vi "Flush Buffer.vi"(8 "error in (no error)":errorcluster, 10 "Wfm Log Instance Index":i32, 11 "Waveform Log in":refnum<class "Waveform Log.lvclass">) -> (0 "error out":errorcluster, 3 "Waveform Log out":refnum<class "Waveform Log.lvclass">)   [LabVIEW 2015, in "Waveform Log.lvclass"]
uses:
  Waveform Log.lvclass
  Waveform Log.lvclass/Waveform Log.ctl
  Buffer/Waveform Buffer/Time Range.ctl
  Buffer/Waveform Buffer/Waveform Buffer.lvclass/Waveform Buffer.ctl
  Waveform Log Wfm Meta Data.ctl
  Buffer/DBL Waveform Buffer/DBL Waveform Buffer.lvclass/DBL Waveform Buffer.ctl
  Logs/Segmented Logs/Segmented Log/Segmented Log.lvclass/Segmented Log.ctl
  Log File Specifications/Log File Specification/Log File Specification.lvclass/Log File Specification.ctl
  Log File Specifications/Waveform TDMS Log File Specification/Waveform TDMS Log File Specification.lvclass/Waveform TDMS Log File Specification.ctl
  Logs/Log Files/Log File/Log File.lvclass/Log File.ctl
  Logs/Log Files/TDMS Log File/TDMS Log File.lvclass/TDMS Log File.ctl
  Logs/Log Files/Text Log File/Text Log File.lvclass/Text Log File.ctl
  Logs/Segmented Logs/Footprint Segmented Log/Footprint Segmented Log.lvclass/Footprint Segmented Log.ctl
  Logs/Segmented Logs/Time Segmented Log/Time Segmented Log.lvclass/Time Segmented Log.ctl
  Buffer/Waveform Buffer/Shift Point by Time.vi
  Buffer/Waveform Buffer/Split Divided Segment.vi
  Buffer/DBL Waveform Buffer/DBL Read from Buffer.vi
  Logs/Segmented Logs/Segmented Log/Write Waveform to Log File Instance.vi
  Buffer/Waveform Buffer/Shift Point by Samples.vi
  Buffer/Waveform Buffer/Get Buffer Length.vi
  Log File Specifications/Log File Specification/Get Log Specification Type.vi
  Log File Specifications/Waveform TDMS Log File Specification/Get Current Group.vi
  Logs/Log Files/Log File/Get Log File Type.vi
  Logs/Log Files/Log File/Write Channel to Log File.vi
  Logs/Log Files/TDMS Log File/Set TDMS Channel Property.vi
  Logs/Log Files/TDMS Log File/Copy Channel Properties.vi
  Logs/Segmented Logs/Segmented Log/Check Close File.vi
  Logs/Segmented Logs/Segmented Log/Check Open File.vi
  Logs/Log Files/TDMS Log File/Write Channel to TDMS Log File.vi
  Logs/Log Files/Text Log File/Write Channel to Text Log File.vi
  Logs/Segmented Logs/Segmented Log/Close Log File Instance.vi
  Logs/Segmented Logs/Segmented Log/Segment Log File.vi
  Logs/Segmented Logs/Segmented Log/Open Log File Instance.vi
  Logs/Log Files/Log File/Close Log File.vi
  Logs/Segmented Logs/Segmented Log/Make File Read-Only.vi
  Logs/Segmented Logs/Segmented Log/On Segmented Log Complete.vi
  Logs/Segmented Logs/Segmented Log/On File Close.vi
  Logs/Segmented Logs/Footprint Segmented Log/Segment Log File (Footprint).vi
  Logs/Segmented Logs/Time Segmented Log/Segment Log File (Time).vi
  Log File Specifications/Log File Specification/Open Log File.vi
  Log File Specifications/Log File Specification/Set Path Tag.vi
  Logs/Segmented Logs/Segmented Log/On File Open.vi
  Log File Specifications/Log File Specification/Set Filename Offset.vi
  Logs/Log Files/TDMS Log File/Close TDMS Log File.vi
  Logs/Log Files/Text Log File/Close Text Log File.vi
  Logs/Segmented Logs/Segmented Log/Get Current Log File Instance.vi
  Logs/Log Files/Log File/Get File Size.vi
  Logs/Log Files/Log File/Get Start Time.vi
  Log File Specifications/Log File Specification/Build File Path.vi
  Log File Specifications/Log File Specification/Resolve File Conflicts.vi
  Shared/Utility/Format File Path for Linux.vi
  <vilib>/Utility/error.llb/Error Cluster From Error Code.vi
  Log File Specifications/Log File Specification/Initialize Log File.vi
  <vilib>/Utility/libraryn.llb/Create Directory Recursive.vi
  <vilib>/Utility/libraryn.llb/Check if File or Folder Exists.vi
  <vilib>/Utility/libraryn.llb/Get File Extension.vi
  Logs/Log Files/Text Log File/Text Log File.lvclass
  Logs/Log Files/TDMS Log File/TDMS Log File.lvclass
  Logs/Log Files/Log File/Log File.lvclass
  Logs/Segmented Logs/Time Segmented Log/Time Segmented Log.lvclass
  Logs/Segmented Logs/Footprint Segmented Log/Footprint Segmented Log.lvclass
  Log File Specifications/Waveform TDMS Log File Specification/Waveform TDMS Log File Specification.lvclass
  Buffer/DBL Waveform Buffer/DBL Waveform Buffer.lvclass
  Buffer/Waveform Buffer/Waveform Buffer.lvclass
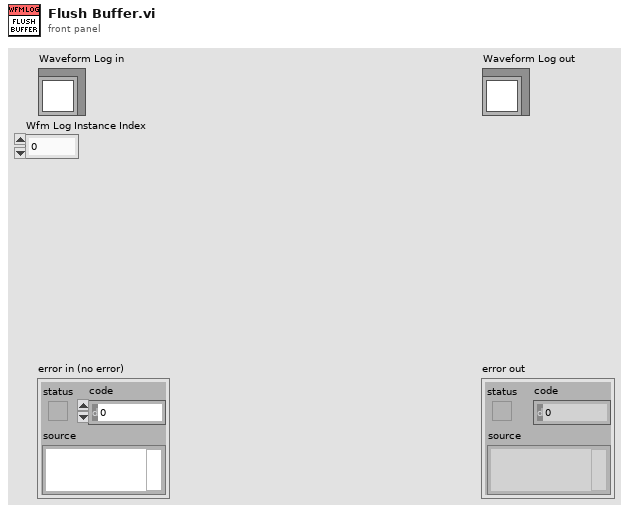
[diagram p1: front panel]
types:
  T1 = typedef "Waveform Buffer.lvclass/Time Range.ctl" = cluster{"Use Receive Time":bool, "Start Time":timestamp, "Stop time":timestamp}
  T2 = typedef "Waveform Log.lvclass/Waveform Log Wfm Meta Data.ctl" = cluster{"Segment ID":u64, "dt":dbl, "t0":timestamp, "tf":timestamp}
  T3 = typedef "Waveform Log.lvclass/Log Instance.ctl" = cluster{"Segmented Log":refnum<data-value>, "Log Waveforms":T4[], "Log Start":timestamp, "Log Stop":timestamp, "Start Trigger Time":timestamp, "Stop Trigger Time":timestamp, "Time of Last Write":timestamp, "Timeout":dbl, "Stop cmd received":bool}
  T4 = typedef "Waveform Log.lvclass/Log Instance Waveform.ctl" = cluster{"Wfm Info":T5, "Count / Instance":i32, "Previous Segment":u64, "Wfm Complete?":bool, "Last Sample Logged":timestamp, "Data Logged":bool, "Log segmented":bool}
  T5 = typedef "Waveform Log.lvclass/Waveform Information.ctl" = cluster{"Name":string, "Wfm Data Type":T6, "Decimation":u32}
  T6 = typedef "Waveform Log.lvclass/Waveform Data Type.ctl" = enum16{"Double", "ComplexDouble"}
  T7 = typedef "Waveform Log.lvclass/Log Waveform.ctl" = cluster{"Buffer Ref":refnum<data-value>, "Wfm Info":T5}
  T8 = typedef "Waveform Buffer.lvclass/Wfm Segment.ctl" = cluster{"ID":u64, "Total samples":i32, "Start":T9, "Finish":T9}
  T9 = typedef "Waveform Buffer.lvclass/Data Point.ctl" = cluster{"Index":i32, "Wfm time":timestamp, "Receive time":timestamp}
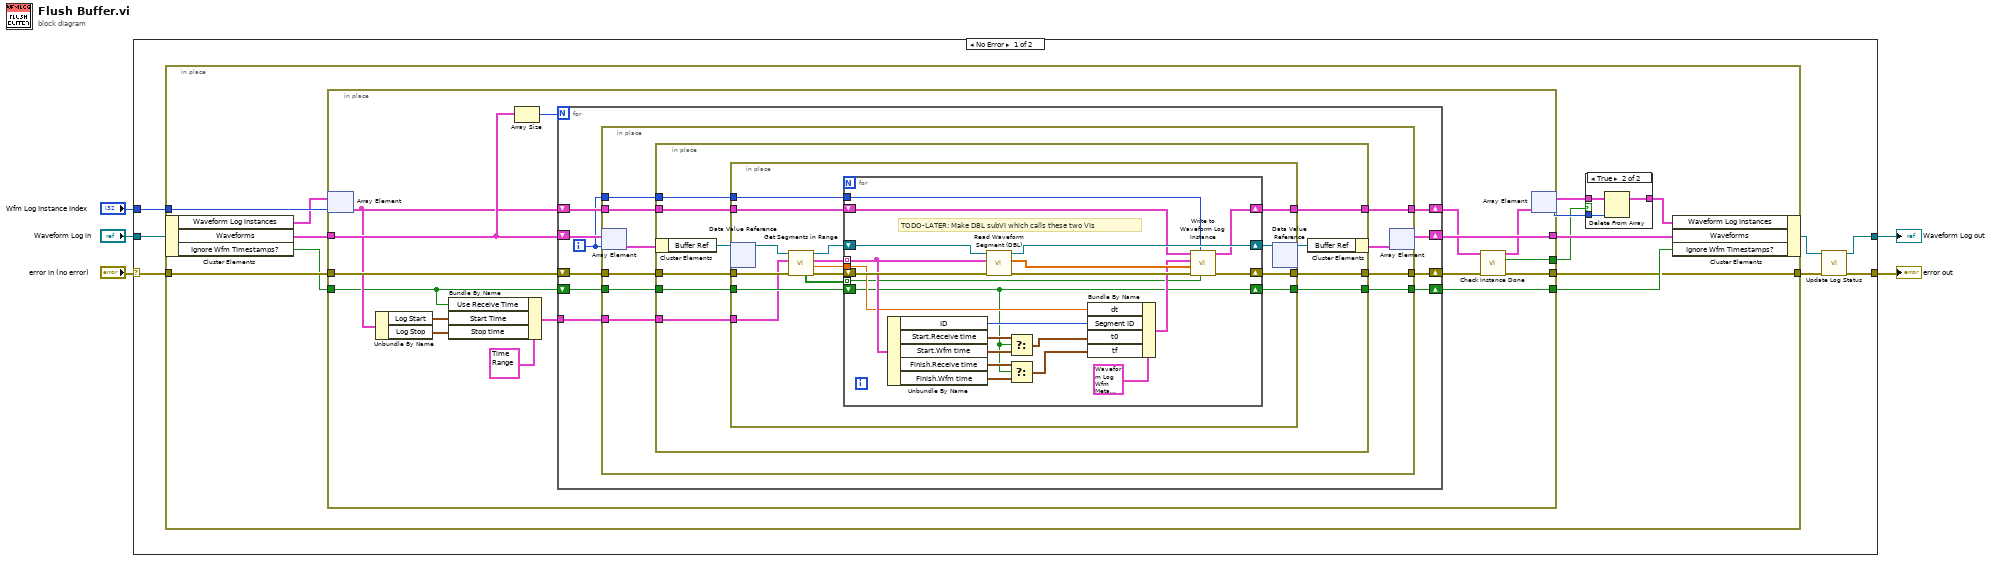
[diagram p0: block diagram]
diagram:
  n1 = case shown="No Error" "error in (no error)" {
    selector: "error in (no error)" -> [w10 w113]
    tunnel: [w6 w113] -> w4
    tunnel: [w7 w112] -> w2
    tunnel: "Waveform Log in" -> [w11 w112]
    tunnel: "Wfm Log Instance Index" -> [w12 _]
    frame No Error {
      n2 = in-place {
        in-place-border: w12 -> [w22]
        in-place-border: w10 -> [w21]
        in-place-border: [w13] -> w9
        n3 = in-place-cluster #1(w11) -> ("Waveform Log Instances"=w20:T3[], "Waveforms"=w24:T7[], "Ignore Wfm Timestamps?"=w19:bool)
        n4 = in-place {
          in-place-border: w24 -> [w44]
          in-place-border: [w43] -> w23
          in-place-border: w21 -> [w42]
          in-place-border: [w31] -> w13
          in-place-border: w19 -> [w35]
          in-place-border: [w36] -> w18
          in-place-border: [w30] -> w14
          n5 = in-place-array #2(w20, w22) -> (w41:T3)
          n6 = Unbundle By Name(w41) -> ("Log Start"=w39:timestamp, "Log Stop"=w38:timestamp)
          n7 = Bundle By Name(cluster=T1 {"Use Receive Time"=FALSE, "Start Time"=timestamp(0 s since 1904-01-01), "Stop time"=timestamp(0 s since 1904-01-01)} ("Time Range"), "Use Receive Time"=w35, "Start Time"=w39, "Stop time"=w38) -> (w37:T1)
          n8 = Array Size(array=w44) -> (size(s)=w29:i32)
          n9 = for {
            N: w29 -> [_]
            shift-right: [w53] -> w43
            shift-left: w44 -> [w54]
            shift-right: [w50] -> w33
            shift-left: w41 -> [w52]
            shift-right: [w48] -> w34
            shift-left: w42 -> [w49]
            tunnel: w37 -> [w46]
            shift-right: [w45] -> w36
            shift-left: w35 -> [w47]
            i -> [w51]
            n10 = in-place {
              in-place-border: w52 -> [w62]
              in-place-border: w51 -> [w61]
              in-place-border: [w60] -> w50
              in-place-border: w49 -> [w59]
              in-place-border: [w58] -> w48
              in-place-border: w47 -> [w57]
              in-place-border: w46 -> [w56]
              in-place-border: [w55] -> w45
              n11 = in-place-array #3(w54, w51) -> (w64:T7)
              n12 = in-place {
                in-place-border: w62 -> [w72]
                in-place-border: w61 -> [w71]
                in-place-border: [w70] -> w60
                in-place-border: w59 -> [w69]
                in-place-border: [w68] -> w58
                in-place-border: w57 -> [w67]
                in-place-border: w56 -> [w66]
                in-place-border: [w65] -> w55
                n13 = in-place-cluster #4(w64) -> ("Buffer Ref"=w74:refnum<data-value>)
                n14 = in-place {
                  in-place-border: w72 -> [w84]
                  in-place-border: w71 -> [w83]
                  in-place-border: [w82] -> w70
                  in-place-border: w69 -> [w80]
                  in-place-border: [w79] -> w68
                  in-place-border: w67 -> [w78]
                  in-place-border: w66 -> [w77]
                  in-place-border: [w76] -> w65
                  n15 = in-place-dvr #5(w74) -> (w86:refnum<class "Waveform Buffer.lvclass">)  [unwired: 1 out]
                  n16 = call "Get Segments in Range.vi"("error in (no error)"=w80, "Time Range"=w77, "Waveform Buffer in"=w86) -> ("error out"=w88:errorcluster, "dt"=w81:dbl, "Wfm Segments"=w89:T8[], "Waveform Buffer out"=w87:refnum<class "Waveform Buffer.lvclass">, "tf Modified?"=w75:bool[])  [unwired: 4 in]
                  n17 = for {
                    tunnel: w89 -> [w103] mode=indexing
                    shift-right: [w109] -> w85
                    shift-left: w87 -> [w110]
                    shift-right: [w106] -> w79
                    shift-left: w88 -> [w111]
                    tunnel: w83 -> [w96]
                    shift-right: [w105] -> w82
                    shift-left: w84 -> [w108]
                    tunnel: w81 -> [w99]
                    shift-right: [w91] -> w76
                    shift-left: w78 -> [w91]
                    tunnel: w75 -> [w90] mode=indexing
                    # "TODO-LATER: Make DBL subVI which calls these two VIs"
                    n18 = Unbundle By Name(w103) -> ("ID"=w102:u64, "Start.Receive time"=w101:timestamp, "Start.Wfm time"=w100:timestamp, "Finish.Receive time"=w94:timestamp, "Finish.Wfm time"=w93:timestamp)
                    n19 = call "Read Waveform Segment (DBL).vi"("error in (no error)"=w111, "Wfm Segment"=w103, "Waveform Buffer in"=w110) -> ("error out"=w107:errorcluster, "Data"=w98:dbl[], "Waveform Buffer out"=w109:refnum<class "Waveform Buffer.lvclass">)  [unwired: 6 in]
                    n20 = Select(t=w101, s=w91, f=w100) -> (s? t:f=w95:timestamp)
                    n21 = Select(t=w94, s=w91, f=w93) -> (s? t:f=w92:timestamp)
                    n22 = Bundle By Name(cluster=T2 {"Segment ID"=0, "dt"=0.0, "t0"=timestamp(0 s since 1904-01-01), "tf"=timestamp(0 s since 1904-01-01)} ("Waveform Data"), "dt"=w99, "Segment ID"=w102, "t0"=w95, "tf"=w92) -> (w97:T2)
                    n23 = call "Write to Waveform Log Instance.vi"("tf Modified?"=w90, "Wfm Index"=w96, "error in (no error)"=w107, "Data"=w98, "Waveform Data"=w97, "Log Instance in"=w108) -> ("error out"=w106:errorcluster, "Log Instance out"=w105:T3)  [unwired: 4 in]
                  }
                  n24 = in-place-dvr #5(w85) -> (w73:refnum<data-value>)  [unwired: 1 out]
                }
                n25 = in-place-cluster #4("Buffer Ref"=w73) -> (w63:T7)
              }
              n26 = in-place-array #3(w63) -> (w53:T7[])  [unwired: 1 out]
            }
          }
          n27 = call "Check Instance Done.vi"("error in (no error)"=w34, "Log Instance in"=w33) -> ("error out"=w31:errorcluster, "Done?"=w30:bool, "Log Instance out"=w32:T3)  [unwired: 7 in]
          n28 = in-place-array #2(w32) -> (w17:T3[], w16:i32)
        }
        n29 = case shown="True" w14 {
          tunnel: w17 -> [w25 w28]
          tunnel: w16 -> [_ w27]
          tunnel: [w25 w26] -> w15
          frame False {
          }
          frame True {
            n30 = Delete From Array(array=w28, index=w27) -> (array with subset deleted=w26:T3[])  [unwired: 1 in, 1 out]
          }
        }
        n31 = in-place-cluster #1("Waveform Log Instances"=w15, "Waveforms"=w23, "Ignore Wfm Timestamps?"=w18) -> (w8:refnum<class "Waveform Log.lvclass">)
      }
      n32 = call "Update Log Status.vi"("error in (no error)"=w9, "Waveform Log in"=w8) -> ("error out"=w6:errorcluster, "Waveform Log out"=w7:refnum<class "Waveform Log.lvclass">)  [unwired: 8 in]
    }
    frame Error {
    }
  }
  "error out" <- w4
  "Waveform Log out" <- w2
